vi "Run Javascript.vi"(6 "Decode Result? (T)":bool=TRUE, 8 "Error In":errorcluster, 9 "Fetch Result? (T)":bool=TRUE, 10 "Javascript in":string, 11 "object in":refnum<class "WebView.lvclass">) -> (0 "Error Out":errorcluster, 2 "Result out":string, 3 "object out":refnum<class "WebView.lvclass">)   [LabVIEW 2024, in "WebView.lvclass"]
uses:
  WebView.lvclass
  <vilib>/sklein/WebView2/Libs/Microsoft.Web.WebView2.Core.dll
  WebView.lvclass/WebView.ctl
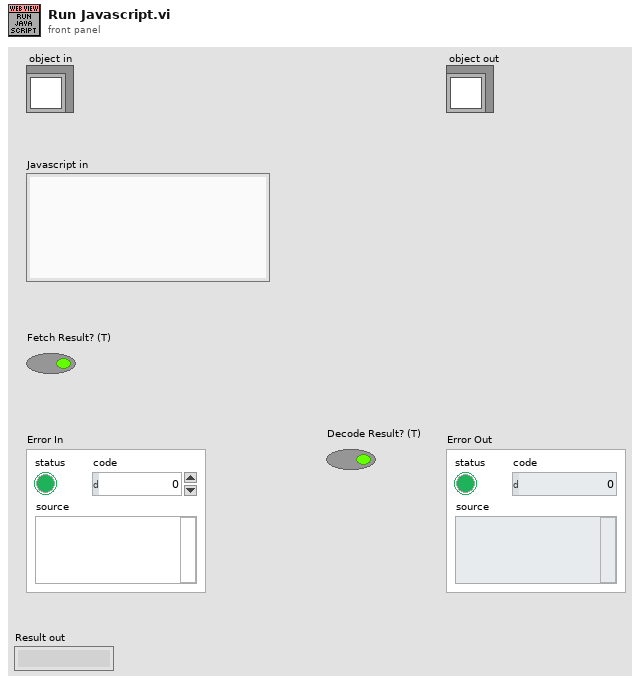
[diagram p1: front panel]
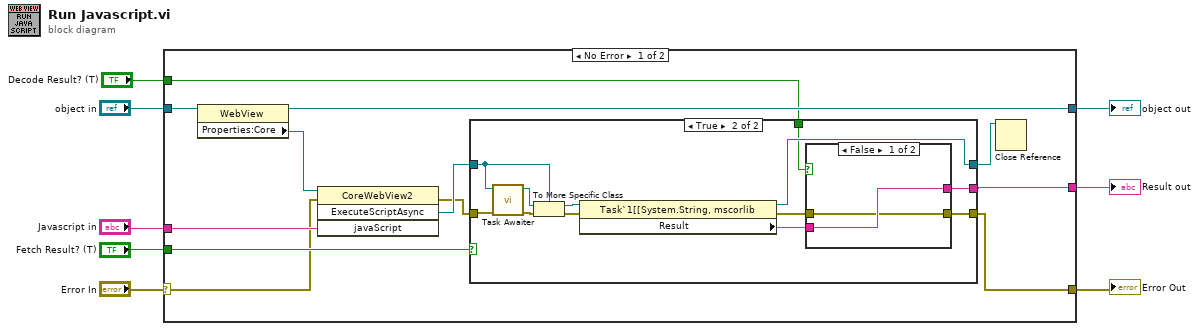
[diagram p0: block diagram]
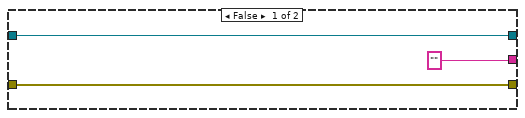
[diagram p2: hidden frame]
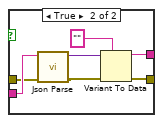
[diagram p3: hidden frame]
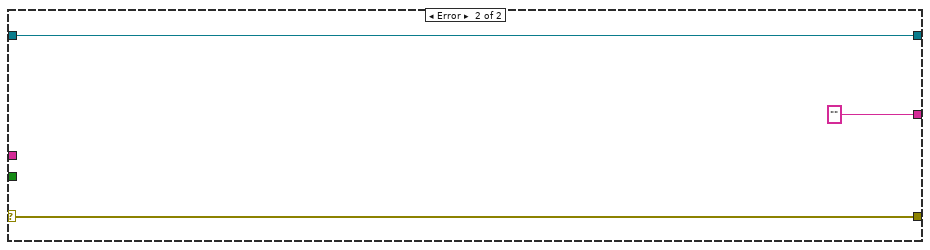
[diagram p4: hidden frame]
diagram:
  n1 = case shown="No Error" "Error In" {
    selector: "Error In" -> [w11 w47]
    tunnel: [w16 w47] -> w7
    tunnel: [w18 w46] -> w5
    tunnel: "object in" -> [w20 w46]
    tunnel: "Javascript in" -> [w12 _]
    tunnel: "Fetch Result? (T)" -> [w17 _]
    tunnel: "Decode Result? (T)" -> [w15 _]
    tunnel: [w14 "" ("Result")] -> w1
    frame No Error {
      n2 = property class="WebView"(reference=w20) -> (reference out=w18:refnum<class "WebView.lvclass">, "Properties:Core"=w13:refnum<k24>)  [unwired: 1 in, 1 out]
      n3 = invoke class="CoreWebView2" method="ExecuteScriptAsync"(reference=w13, error in=w11, "javaScript"=w12) -> (error out=w9:errorcluster, "ExecuteScriptAsync"=w10:refnum<k24>)  [unwired: 1 in, 2 out]
      n4 = case shown="True" w17 {
        tunnel: w10 -> [w22 w25]
        tunnel: w9 -> [w23 w28]
        tunnel: [w22 w35] -> w19
        tunnel: ["" ("Result") w34] -> w14
        tunnel: [w23 w33] -> w16
        tunnel: w15 -> [_ w24]
        frame False {
        }
        frame True {
          n5 = call "Task Awaiter.vi"("error in (no error)"=w28, "Task"=w25) -> ("error out"=w27:errorcluster, "Task"=w26:refnum<k24>)  [unwired: 7 in, 1 out]
          n6 = To More Specific Class(target class=w25, reference=w26, error in=w27) -> (specific class reference=w29:refnum<k24>, error out=w30:errorcluster)
          n7 = property class="Task`1[[System.String, mscorlib"(reference=w29, error in=w30) -> (reference out=w35:refnum<k24>, error out=w32:errorcluster, "Result"=w31:string)
          n8 = case shown="False" w24 {
            tunnel: [w37 w43] -> w34
            tunnel: [w36 w42] -> w33
            tunnel: w32 -> [w36 w40]
            tunnel: w31 -> [w37 w41]
            frame False {
            }
            frame True {
              n9 = call "Json Parse.vi"("error in (no error)"=w40, "JSON in"=w41) -> ("error out"=w39:errorcluster, "variant"=w38:variant)  [unwired: 8 in]
              n10 = Variant To Data(error in=w39, type="", Variant=w38) -> (data=w43:string, error out=w42:errorcluster)
            }
          }
        }
      }
      n11 = Close Reference(reference=w19) -> ()  [unwired: 1 in, 1 out]
    }
    frame Error {
    }
  }
  "Error Out" <- w7
  "object out" <- w5
  "Result out" <- w1
